vi "DeleteFromComboBox(SubVI).vi"(1 "Index":dbl, 2 "Array In":cluster{"String":string, "Value":string}[](array[cluster])) -> (0 "Array Out":cluster{"String":string, "Value":string}[](array[cluster]))   [LabVIEW 2018]
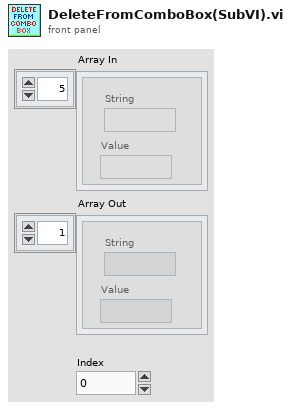
[diagram p1: front panel]
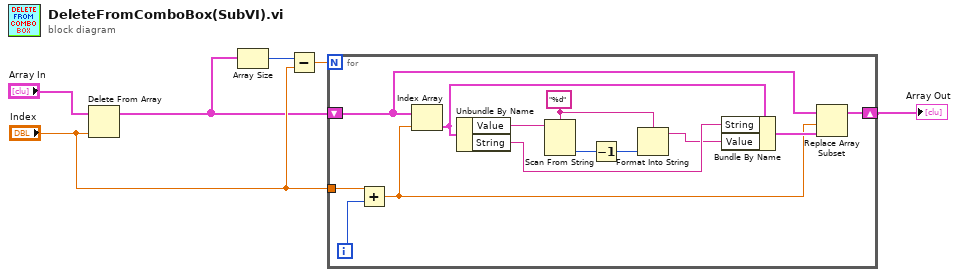
[diagram p0: block diagram]
diagram:
  n1 = Delete From Array(array="Array In", index="Index") -> (array with subset deleted=w1:cluster{"String":string, "Value":string}[])  [unwired: 1 in, 1 out]
  n2 = Array Size(array=w1) -> (size(s)=w6:i32)
  n3 = Subtract(x=w6, y="Index") -> (x-y=w5:dbl)
  n4 = for {
    N: w5 -> [_]
    shift-right: [w10] -> w3
    shift-left: w1 -> [w14]
    tunnel: "Index" -> [w9]
    i -> [w8]
    w16 = "%d" ("format string")
    n5 = Add(x=w9, y=w8) -> (x+y=w7:dbl)
    n6 = Index Array(array=w14, index=w7) -> (element=w15:cluster{"String":string, "Value":string})
    n7 = Unbundle By Name(w15) -> ("Value"=w19:string, "String"=w13:string)
    n8 = Scan From String(format string=w16, input string=w19) -> (output 1=w18:i32)  [unwired: 3 in, 3 out]
    n9 = Decrement(x=w18) -> (x-1=w17:i32)
    n10 = Format Into String(format string=w16, w17) -> (resulting string=w12:string)  [unwired: 2 in, 1 out]
    n11 = Bundle By Name(cluster=w15, "String"=w13, "Value"=w12) -> (w11:cluster{"String":string, "Value":string})
    n12 = Replace Array Subset(array=w14, new element=w11, index=w7) -> (w10:cluster{"String":string, "Value":string}[])
  }
  "Array Out" <- w3
